vi "erasewater.vi"(10 "GIC Input":T1={"Real/Sim"=FALSE, "WP Lats and Longs"={"WP Lats"=[], "WP Longs"=[]}, "GPS Time Int"=0.0, "GPS Com Port"="", "Compass Com Port"="", "Prop Com Port"="", "GPS Data"=[], "Compass"=0.0, "LMS Vector"=[], "Vision Vector"=[], "Direction Cmd"=0.0, "Speed Cmd"=0.0, "Time of Last GPS"=0.0, "WP Vector"=[], "WP Number"=0, "Num of WPs"=0, "SW Map"=[], "Obst Lats and Longs"={"Obst Lats"=[], "Obst Longs"=[]}, "Parameters"=[], "Path Cluster"={"Path x nodes"=[], "Path y nodes"=[]}, "     Use ?\nOff       On"=[TRUE, TRUE, FALSE, FALSE]} {"Obst Lats and Longs"."Obst Longs" format="%#_8g"; "Obst Lats and Longs"."Obst Lats" format="%#_8g"}) -> (2 "GIC Output":T1={"Real/Sim"=FALSE, "WP Lats and Longs"={"WP Lats"=[], "WP Longs"=[]}, "GPS Time Int"=0.0, "GPS Com Port"="", "Compass Com Port"="", "Prop Com Port"="", "GPS Data"=[], "Compass"=0.0, "LMS Vector"=[], "Vision Vector"=[], "Direction Cmd"=0.0, "Speed Cmd"=0.0, "Time of Last GPS"=0.0, "WP Vector"=[], "WP Number"=0, "Num of WPs"=0, "SW Map"=[], "Obst Lats and Longs"={"Obst Lats"=[], "Obst Longs"=[]}, "Parameters"=[], "Path Cluster"={"Path x nodes"=[], "Path y nodes"=[]}, "     Use ?\nOff       On"=[TRUE, TRUE, FALSE, FALSE]} {"Obst Lats and Longs"."Obst Longs" format="%#_8g"; "Obst Lats and Longs"."Obst Lats" format="%#_8g"})   [LabVIEW 2014]
panel:
  out "test3":dbl
  out "Test2":dbl
  in  "Test Parameters":dbl[](array[numeric])
  out "Numeric":dbl
  # "WaterFall"
  # "GPS"
  # "LMS"
  # "Vision"
  # "Prop"
  # "GPS"
  # "LMS"
  # "Vision"
  # "Prop"
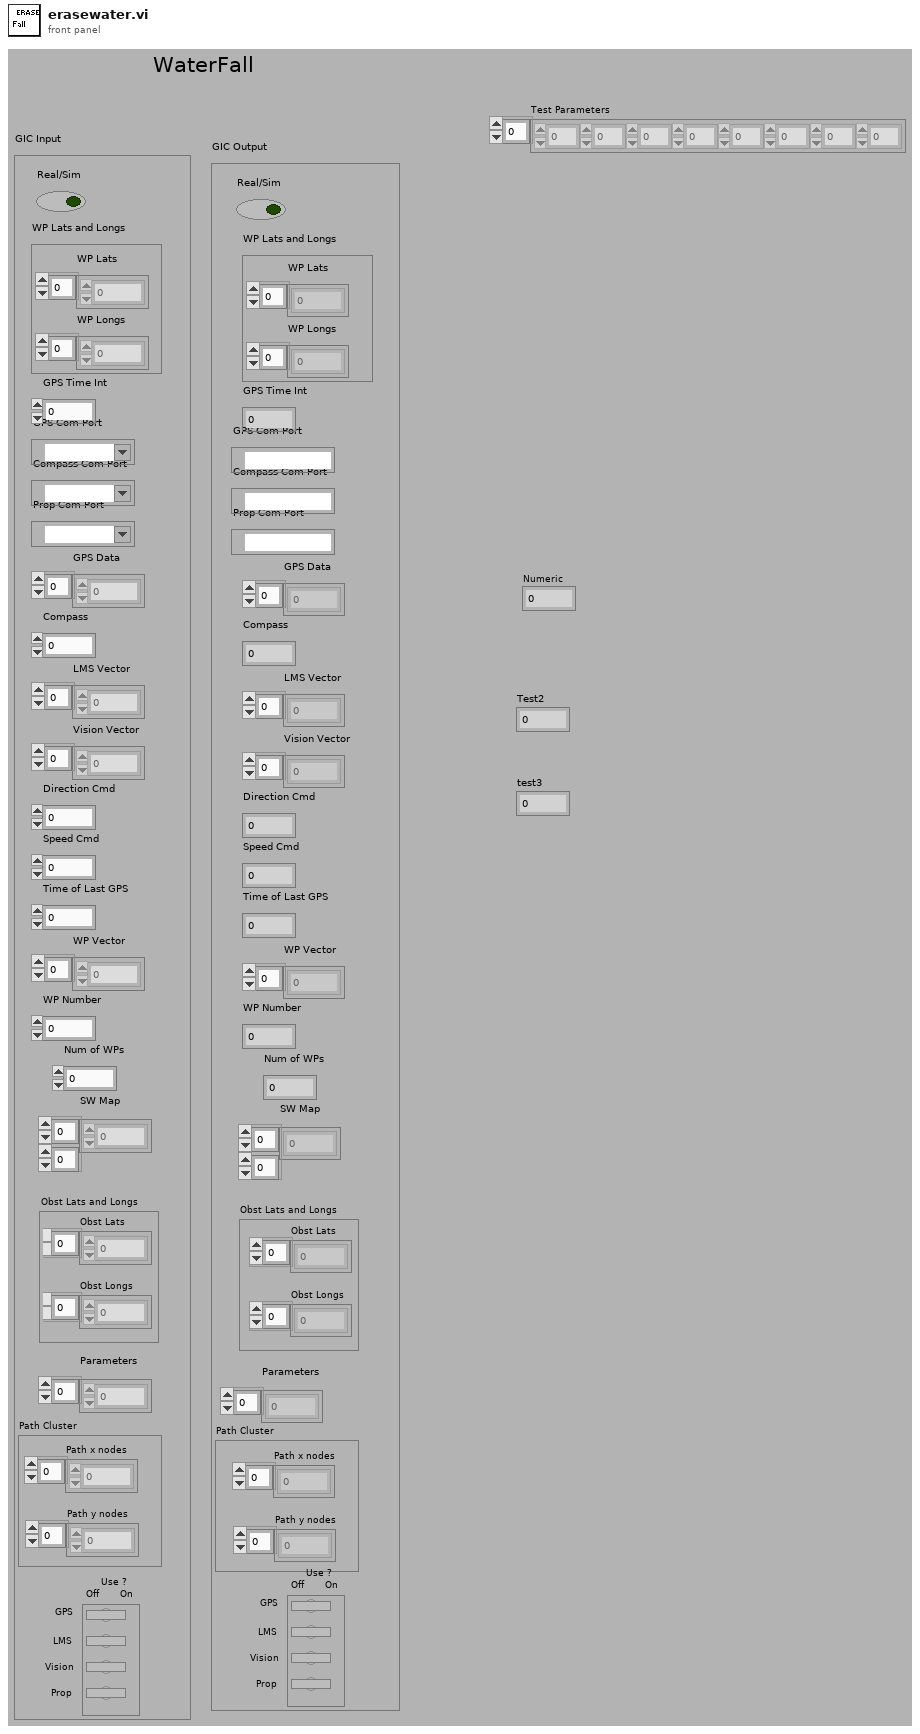
[diagram p1: front panel]
types:
  T1 = cluster{"Real/Sim":bool, "WP Lats and Longs":cluster{"WP Lats":dbl[], "WP Longs":dbl[]}, "GPS Time Int":dbl, "GPS Com Port":refnum<visa-resource-name>, "Compass Com Port":refnum<visa-resource-name>, "Prop Com Port":refnum<visa-resource-name>, "GPS Data":dbl[], "Compass":dbl, "LMS Vector":dbl[], "Vision Vector":dbl[], "Direction Cmd":dbl, "Speed Cmd":dbl, "Time of Last GPS":dbl, "WP Vector":dbl[], "WP Number":i32, "Num of WPs":i16, "SW Map":i32[][], "Obst Lats and Longs":cluster{"Obst Lats":dbl[], "Obst Longs":dbl[]}, "Parameters":dbl[], "Path Cluster":cluster{"Path x nodes":dbl[], "Path y nodes":dbl[]}, "     Use ?\nOff       On":bool[]}
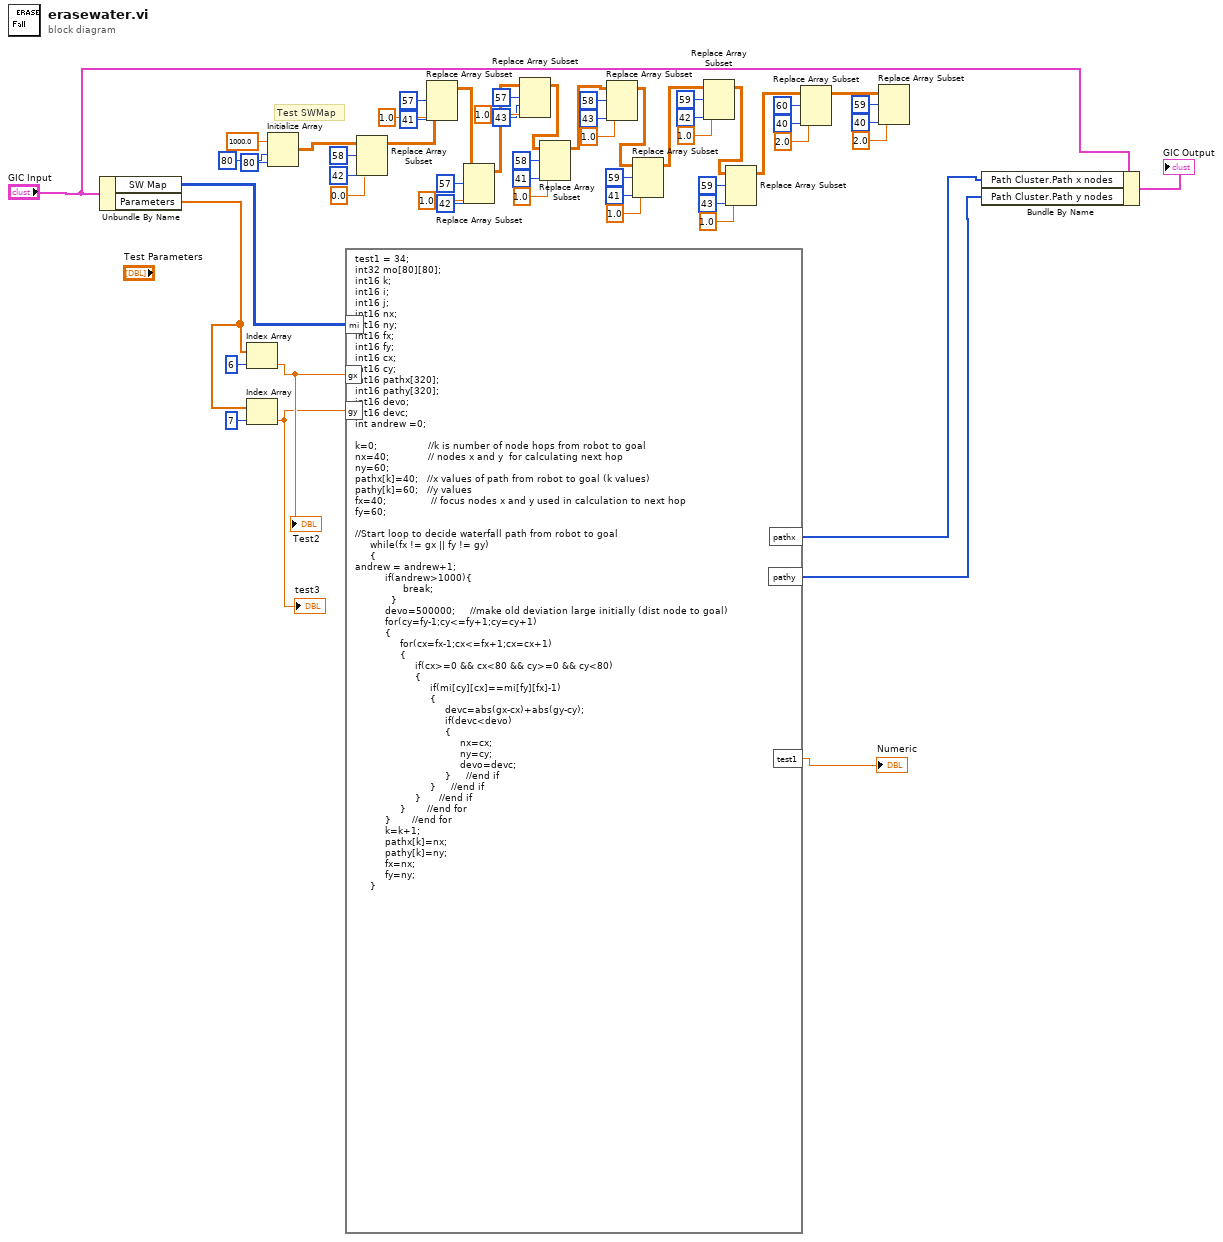
[diagram p0: block diagram]
diagram:
  # "Test SWMap"
  n1 = Unbundle By Name("GIC Input") -> ("SW Map"=w38:i32[][], "Parameters"=w39:dbl[])
  n2 = Index Array(array=w39, index=6) -> (element=w2:dbl)
  "Test2" <- w2
  n3 = Index Array(array=w39, index=7) -> (element=w1:dbl)
  "test3" <- w1
  n4 = Initialize Array(1000.0 ("element"), 80 ("dimension size"), 80 ("dimension size")) -> (w55:dbl[][])
  n5 = formula code="test1 = 34;\nint32 mo[80][80];\nint16 k;\nint16 i;\nint16 j;\nint16 nx;\nint16 ny;\nint16 fx;\nint16 fy;\nint16 cx;\nint16 cy;\nint16 pathx[320];\nint16 pathy[320];\nint16 devo;\nint16 devc;\nint andrew =0;\n\nk=0;                 //k is number of node hops from robot to goal\nnx=40;             // nodes x and y  for calculating next hop\nny=60;\npathx[k]=40;   //x values of path from robot to goal (k values)\npathy[k]=60;   //y values\nfx=40;               // focus nodes x and y used in calculation to next hop\nfy=60;\n\n//Start loop to decide waterfall path from robot to goal\n     while(fx != gx || fy != gy)\n     {\nandrew = andrew+1;\n          if(andrew>1000){\n                break;\n            }\n          devo=500000;     //make old deviation large initially (dist node to goal)\n          for(cy=fy-1;cy<=fy+1;cy=cy+1)\n          {\n               for(cx=fx-1;cx<=fx+1;cx=cx+1)\n               {\n                    if(cx>=0 && cx<80 && cy>=0 && cy<80)\n                    {\n                         if(mi[cy][cx]==mi[fy][fx]-1)\n                         {\n                              devc=abs(gx-cx)+abs(gy-cy);\n                              if(devc<devo)\n                              {\n                                   nx=cx;\n                                   ny=cy;\n                                   devo=devc;\n                              }     //end if\n                         }     //end if\n                    }      //end if\n               }       //end for\n          }       //end for\n          k=k+1;\n          pathx[k]=nx;\n          pathy[k]=ny;\n          fx=nx;\n          fy=ny;\n     }"("mi"=w38, "gx"=w2, "gy"=w1) -> ("test1"=→"Numeric":dbl, "pathx"=w37:i16[], "pathy"=w36:i16[])
  n6 = Replace Array Subset(array=w55, new element=0.0 ("new element/subarray"), index (row)=58, index (col)=42 ("disabled index (col)")) -> (w51:dbl[][])
  n7 = Replace Array Subset(array=w51, new element=1.0 ("new element/subarray"), index (row)=57, index (col)=41 ("disabled index (col)")) -> (w47:dbl[][])
  n8 = Replace Array Subset(array=w47, new element=1.0 ("new element/subarray"), index (row)=57, index (col)=42 ("disabled index (col)")) -> (w35:dbl[][])
  n9 = Replace Array Subset(array=w35, new element=1.0 ("new element/subarray"), index (row)=57, index (col)=43 ("disabled index (col)")) -> (w31:dbl[][])
  n10 = Replace Array Subset(array=w31, new element=1.0 ("new element/subarray"), index (row)=58, index (col)=41 ("disabled index (col)")) -> (w27:dbl[][])
  n11 = Replace Array Subset(array=w27, new element=1.0 ("new element/subarray"), index (row)=58, index (col)=43 ("disabled index (col)")) -> (w23:dbl[][])
  n12 = Replace Array Subset(array=w23, new element=1.0 ("new element/subarray"), index (row)=59, index (col)=41 ("disabled index (col)")) -> (w19:dbl[][])
  n13 = Replace Array Subset(array=w19, new element=1.0 ("new element/subarray"), index (row)=59, index (col)=42 ("disabled index (col)")) -> (w15:dbl[][])
  n14 = Replace Array Subset(array=w15, new element=1.0 ("new element/subarray"), index (row)=59, index (col)=43 ("disabled index (col)")) -> (w11:dbl[][])
  n15 = Replace Array Subset(array=w11, new element=2.0 ("new element/subarray"), index (row)=60, index (col)=40 ("disabled index (col)")) -> (w7:dbl[][])
  n16 = Replace Array Subset(array=w7, new element=2.0 ("new element/subarray"), index (row)=59, index (col)=40 ("disabled index (col)")) -> ()  [unwired: 1 out]
  n17 = Bundle By Name(cluster="GIC Input", "Path Cluster.Path x nodes"=w37, "Path Cluster.Path y nodes"=w36) -> (→"GIC Output":T1)
